vi "Eat.vi"(8 "error in (no error)":errorcluster, 11 "Hungry Hippo In":refnum<class "Hungry Hippo.lvclass">) -> (0 "error out":errorcluster, 2 "Result":string, 3 "Hungry Hippo Out":refnum<class "Hungry Hippo.lvclass">)   [LabVIEW 2020, in "Hungry Hippo.lvclass"]
uses:
  Hungry Hippo.lvclass
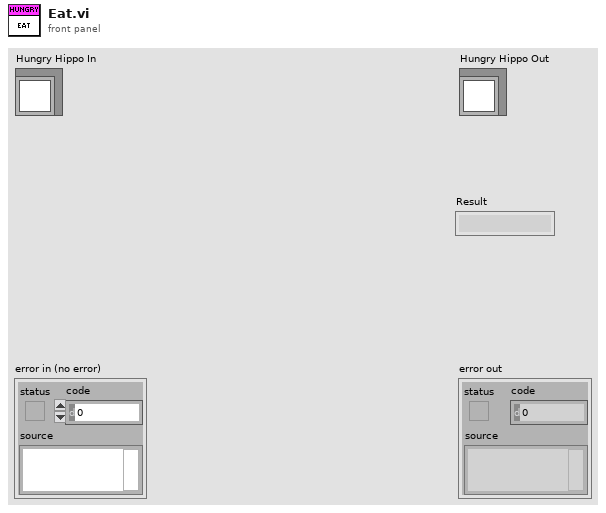
[diagram p1: front panel]
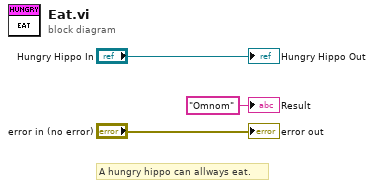
[diagram p0: block diagram]
diagram:
  # "A hungry hippo can allways eat."
  "error out" <- "error in (no error)"
  "Hungry Hippo Out" <- "Hungry Hippo In"
  "Result" <- "Omnom" ("Result")
